vi "API_Reference_List.vi"(1 "API Function Array In":cluster{string, "VI Reference":refnum<vi>}[](array[cluster]), 2 "Command Sequence":cluster{string, string[], dbl[], dbl}[](array[cluster])) -> (0 "API Function Array Out":cluster{string, "VI Reference":refnum<vi>}[](array[cluster]))   [LabVIEW 2011]
doc: "This VI examines the supplied command sequence, creates the necessary polymorphic API VI references, and appends them to the API Function Array. This code is used when a new growth sequence file is opened in the editor. When a new file is opened, no API VI references have been created in memory,necessitating the use of this VI."
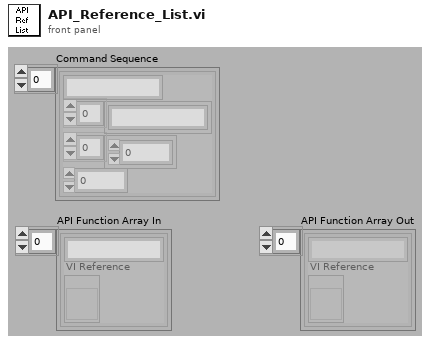
[diagram p1: front panel]
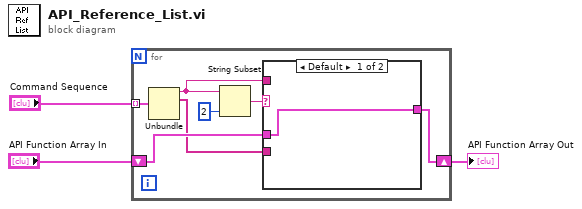
[diagram p0: block diagram]
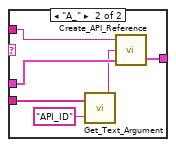
[diagram p2: hidden frame]
diagram:
  n1 = for {
    tunnel: "Command Sequence" -> [w10] mode=indexing
    shift-right: [w7] -> w3
    shift-left: "API Function Array In" -> [w9]
    n2 = Unbundle(w10) -> (w6:string, w8:string[])  [unwired: 2 out]
    n3 = String Subset(string=w6, length (rest)=2 ("length (rest)")) -> (substring=w4:string)  [unwired: 1 in]
    n4 = case shown="Default" w4 {
      tunnel: w6 -> [_ w17]
      tunnel: w9 -> [w11 w16]
      tunnel: [w11 w15] -> w7
      tunnel: w8 -> [_ w14]
      frame Default {
      }
      frame "A_" {
        n5 = call "Get_Text_Argument.vi"("Argument"="API_ID", "Argument List"=w14) -> ("Text"=w12:string)
        n6 = call "Create_API_Reference.vi"("API Function Array In"=w16, "ID"=w12, "Command"=w17) -> ("API Function Array Out"=w15:cluster{string, "VI Reference":refnum<vi>}[])  [unwired: 1 out]
      }
    }
  }
  "API Function Array Out" <- w3
